vi "Initialize Hardware References.vi"(8 "error in (no error)":errorcluster, 11 "Hardware Resources in":T1) -> (0 "error out":errorcluster, 3 "Hardware Resources out":T1)   [LabVIEW 2022 SP3, in "Acquisition.lvlib"]
doc: "Initialize the hardware references."
uses:
  Acquisition.lvlib
  Network Configuration.ctl
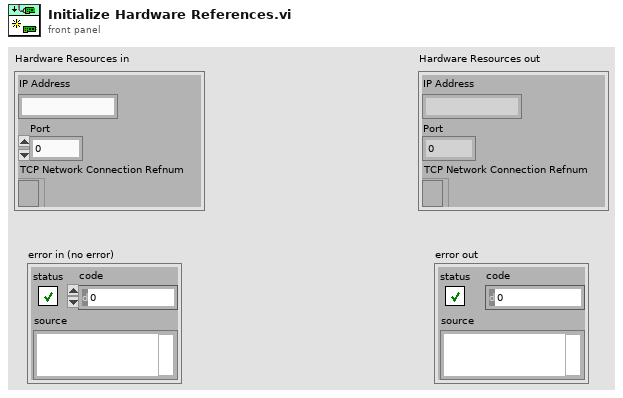
[diagram p1: front panel]
types:
  T1 = typedef "Acquisition.lvlib/Network Configuration.ctl" = cluster{"IP Address":string, "Port":dbl, "TCP Network Connection Refnum":refnum<k5>}
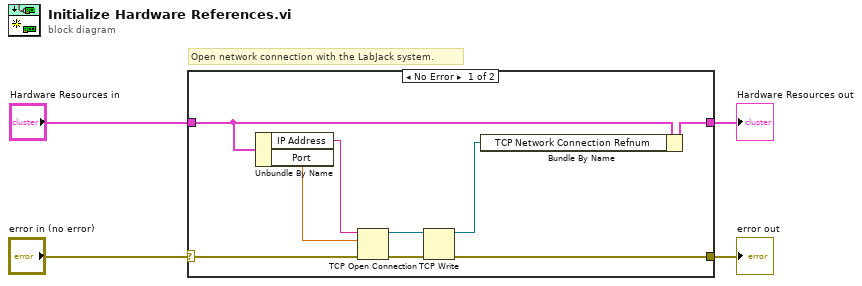
[diagram p0: block diagram]
diagram:
  # "Open network connection with the LabJack system."
  n1 = case shown="No Error" "error in (no error)" {
    selector: "error in (no error)" -> [w12 w14]
    tunnel: [w11 w14] -> w3
    tunnel: "Hardware Resources in" -> [w7 w15]
    tunnel: [w6 w15] -> w1
    frame No Error {
      n2 = Unbundle By Name(w7) -> ("IP Address"=w9:string, "Port"=w8:dbl)
      n3 = TCP Open Connection(address=w9, remote port or service name=w8, error in (no error)=w12) -> (connection ID=w10:refnum<k5>, error out=w13:errorcluster)  [unwired: 2 in]
      n4 = TCP Write(connection ID=w10, error in (no error)=w13) -> (connection ID out=w5:refnum<k5>, error out=w11:errorcluster)  [unwired: 2 in, 1 out]
      n5 = Bundle By Name(cluster=w7, "TCP Network Connection Refnum"=w5) -> (w6:T1)
    }
    frame Error {
    }
  }
  "Hardware Resources out" <- w1
  "error out" <- w3
